vi "总磷流程.vi"   [LabVIEW 2016]
types:
  T1 = enum16{"步骤1", "步骤2", "步骤3", "步骤4", "步骤5", "步骤6", "步骤7", "步骤8", "步骤9", "步骤10"}
  T2 = enum32{"Bad", "Idle", "Run top level", "Running"}
  T3 = cluster{"因子编码":u32, "单位":u16, "标样参考值":sgl, "水样数据时间":timestamp, "水样实测值":sgl, "水样数据标识":string, "标样数据时间":timestamp, "标样实测值":sgl, "标样数据标识":string, "空白数据时间":timestamp, "空白实测值":sgl, "空白数据标识":string, "零点核查数据时间":timestamp, "零点核查实测值":sgl, "零点核查数据标识":string, "跨度核查数据时间":timestamp, "跨度核查实测值":sgl, "跨度核查数据标识":string, "加标回收数据时间":timestamp, "加标回收实测值":sgl, "加标回收数据标识":string, "平行样数据时间":timestamp, "平行样实测值":sgl, "平行样数据标识":string}
  T4 = cluster{"系统时间":timestamp, "工作状态":u16, "测量模式":u16, "告警代码":enum16{"无告警", "缺试剂告警", "缺水样告警", "缺蒸馏水告警", "缺标液告警", "仪表漏液告警", "标定异常告警", "超量程告警", "加热异常", "低试剂预警", "超上限告警", "超下限告警", "仪表内部其他异常", "滴定异常告警", "电极异常告警", "量程切换告警", "参数设置告警", "PH电极电位异常", "电导率电极异常", "浊度光度异常", "溶解氧电极异常", "溶解氧光强异常", "温度异常告警", "PH异常告警", "溶解氧异常告警", "电导率异常告警", "浊度异常告警", "叶绿素异常告警", "藻密度异常告警", "蓝绿藻异常告警", "ORP异常告警", "氨氮异常告警", "清洁刷异常告警", "SD卡异常告警", "蓝牙异常告警", "Wifi异常告警", "流程异常告警"}, "故障代码":enum16{"无故障", "电机故障", "温度故障", "通讯故障", "滴定故障"}, "日志代码":u16, "软件版本":u16, "F0":sgl, "F1":sgl, "F2":sgl, "F3":sgl, "T":sgl, "H":sgl, "id":u16, "flowid":u16, "量程":u16}
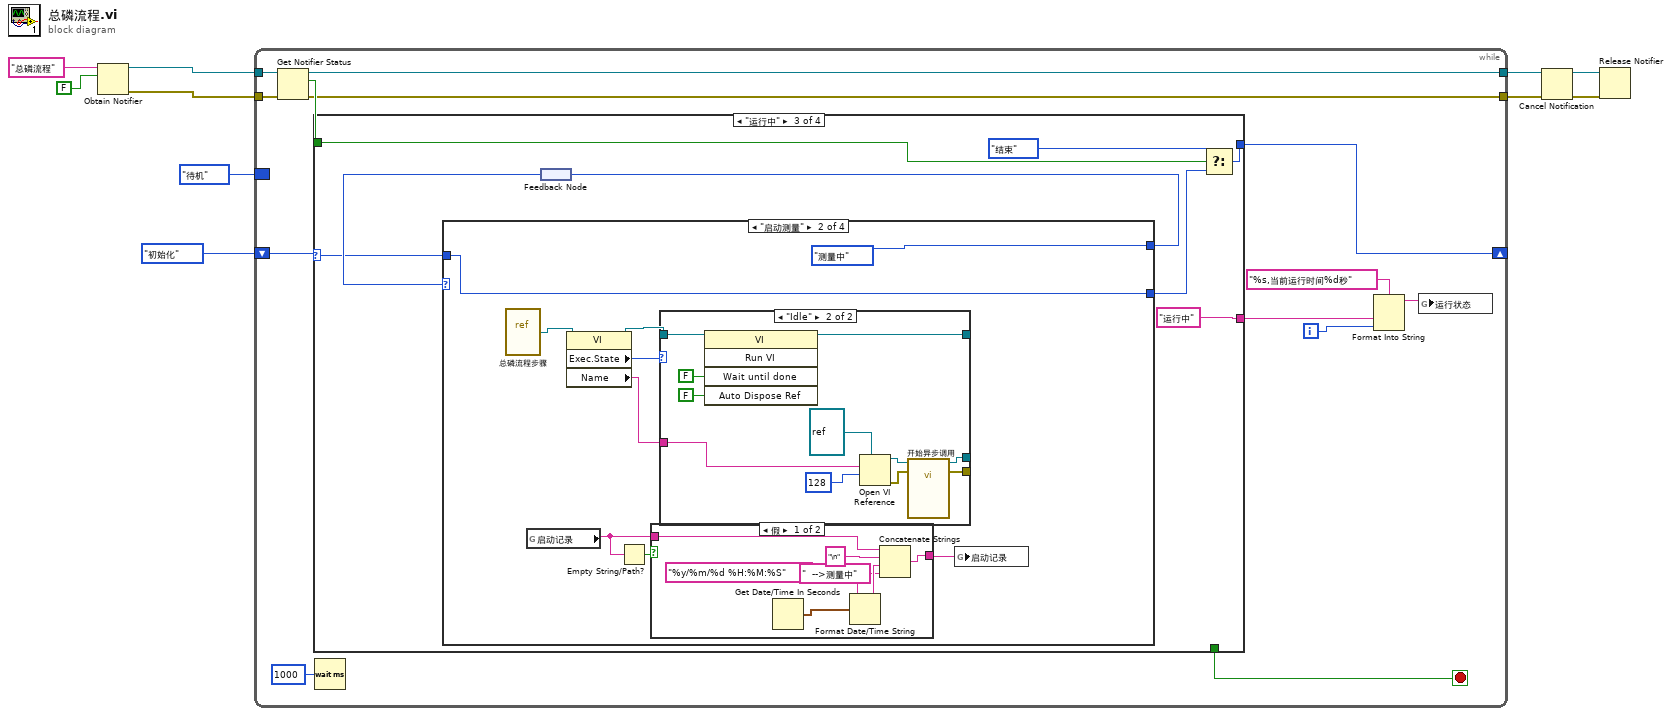
[diagram p0: block diagram]
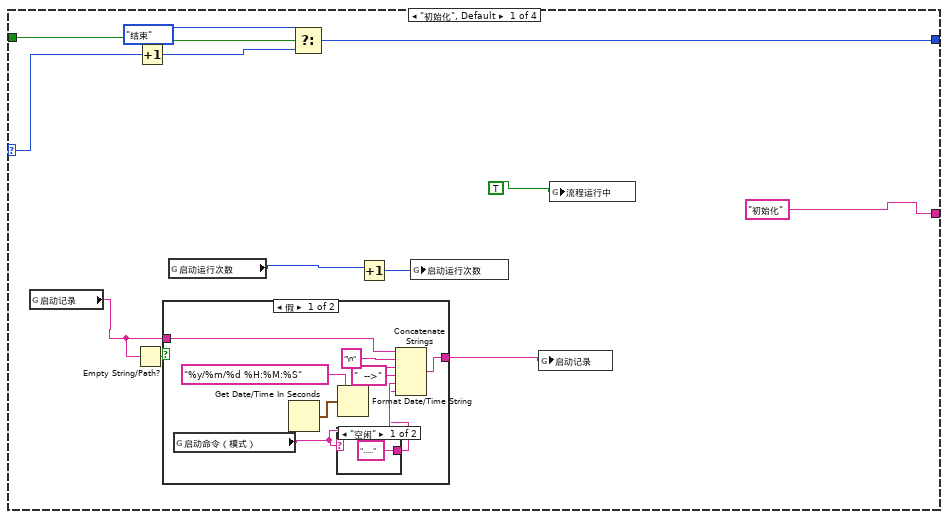
[diagram p2: hidden frame]
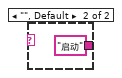
[diagram p3: hidden frame]
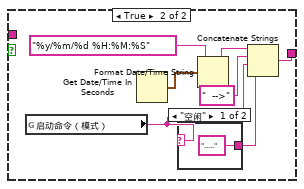
[diagram p4: hidden frame]
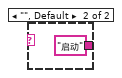
[diagram p5: hidden frame]
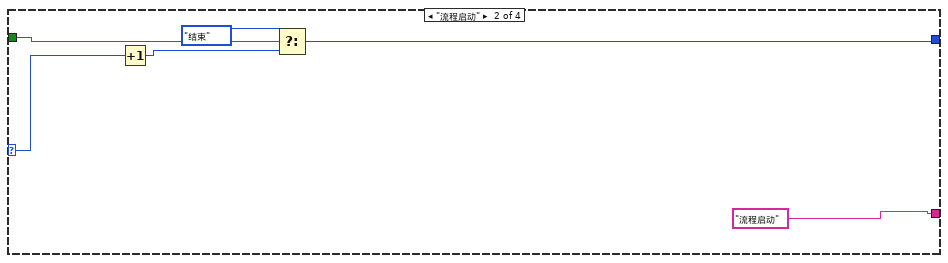
[diagram p6: hidden frame]
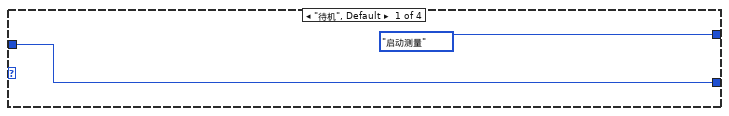
[diagram p7: hidden frame]
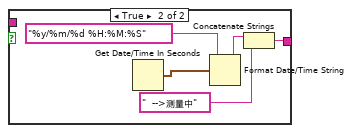
[diagram p8: hidden frame]
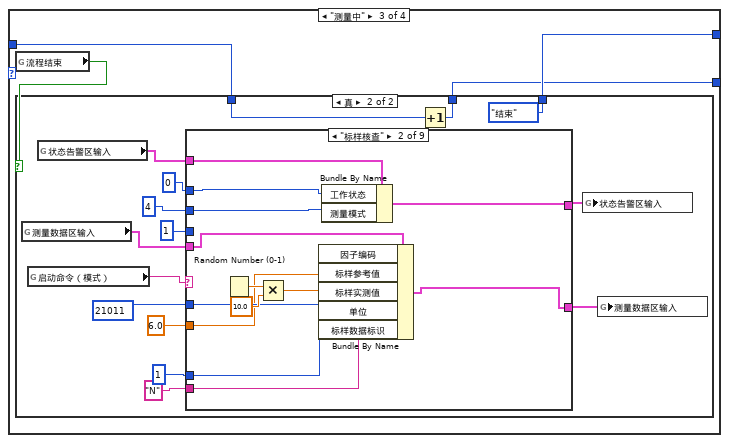
[diagram p10: hidden frame]
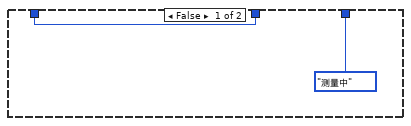
[diagram p11: hidden frame]
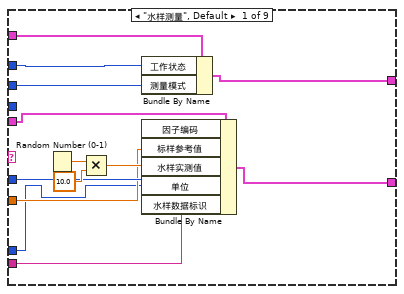
[diagram p12: hidden frame]
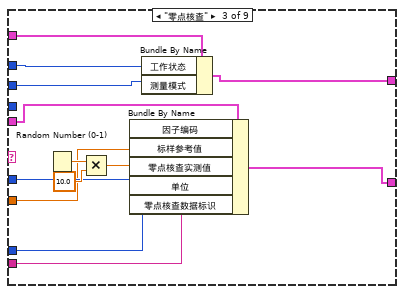
[diagram p13: hidden frame]
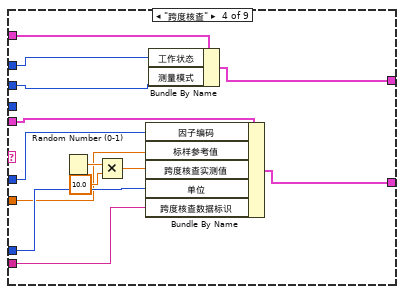
[diagram p14: hidden frame]
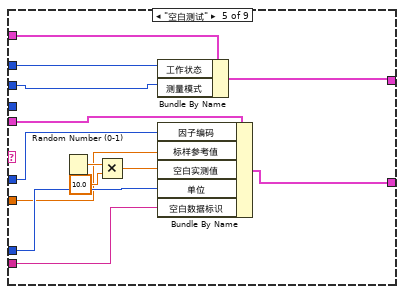
[diagram p15: hidden frame]
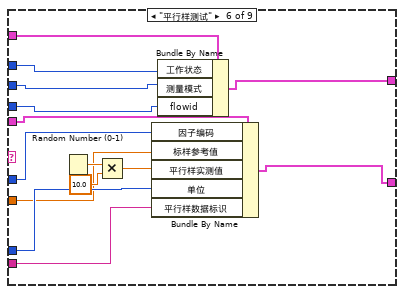
[diagram p16: hidden frame]
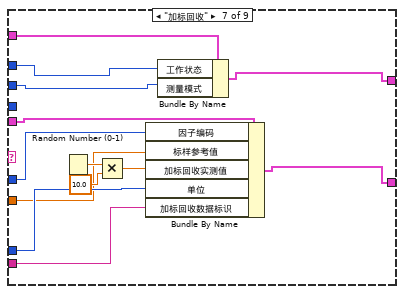
[diagram p17: hidden frame]
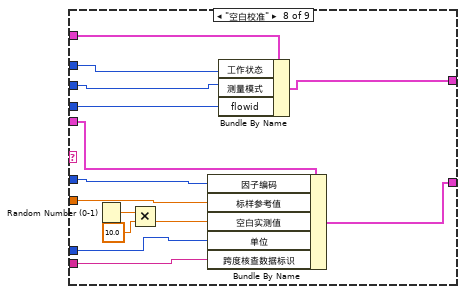
[diagram p18: hidden frame]
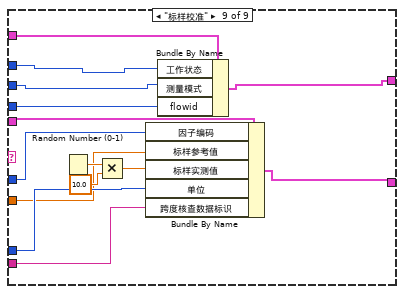
[diagram p19: hidden frame]
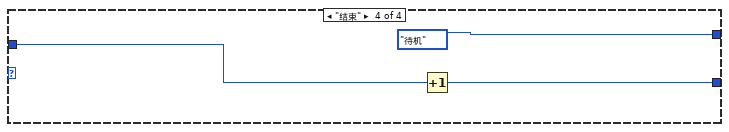
[diagram p20: hidden frame]
diagram:
  n1 = Obtain Notifier(name (unnamed)="总磷流程" ("名称（未命名）"), notification data type=FALSE) -> (notifier out=w7:refnum<notifier>, error out=w6:errorcluster)  [unwired: 2 in, 1 out]
  n2 = while {
    shift-right: [w20] -> _
    shift-left: enum16{"初始化", "流程启动", "运行中", "结束"}."初始化" ("枚举") -> [w23]
    tunnel: w7 -> [w15]
    tunnel: w6 -> [w14]
    tunnel: [w13] -> w5
    tunnel: [w12] -> w4
    border: enum16{"待机", "启动测量", "测量中", "结束"}."待机" -> [_]
    i -> [w18]
    stop <- w16 stop-if-true
    n3 = Get Notifier Status(notifier=w15, error in (no error)=w14) -> (notifier out=w13:refnum<notifier>, current notification=w21:bool, error out=w12:errorcluster)  [unwired: 2 out]
    n4 = case shown="\"运行中\"" w23 {
      selector: w23 -> [w33 w58 w64 w255]
      tunnel: [_ _ _ TRUE ("x")] -> w16
      tunnel: w21 -> [w35 w59 w68 _]
      tunnel: [w31 w57 w63 w255] -> w20
      tunnel: ["初始化" ("输入 1") "流程启动" ("输入 1") "运行中" ("输入 1") "结束" ("输入 1")] -> w17
      frame "初始化", Default {
        n5 = global read "总磷全局.vi" "启动记录"() -> (w25:string)
        n6 = Empty String/Path?(string/path=w25) -> (empty?=w29:bool)
        n7 = Increment(x=w33) -> (x+1=w32:enum16{"初始化", "流程启动", "运行中", "结束"})
        n8 = case shown="假" w29 {
          tunnel: w25 -> [w44 _]
          tunnel: [w39 w50] -> w24
          frame False {
            n9 = global read "总磷全局.vi" "启动命令（模式）"() -> (w37:string)
            n10 = Get Date/Time In Seconds() -> (seconds since 1Jan1904=w42:timestamp)
            n11 = case shown="\"空闲\"" w37 {
              tunnel: ["....." ("字符串") "启动" ("字符串")] -> w36
              frame "空闲" {
              }
              frame "", Default {
              }
            }
            n12 = Format Date/Time String(time format string (%c)="%y/%m/%d %H:%M:%S" ("时间格式字符串(%c)"), seconds (now)=w42) -> (date/time string=w40:string)  [unwired: 1 in]
            n13 = Concatenate Strings(w44, "\n" ("字符串"), w40, "  -->" ("字符串"), w37, w36) -> (w39:string)
          }
          frame True {
            n14 = global read "总磷全局.vi" "启动命令（模式）"() -> (w48:string)
            n15 = Get Date/Time In Seconds() -> (seconds since 1Jan1904=w53:timestamp)
            n16 = case shown="\"空闲\"" w48 {
              tunnel: ["....." ("字符串") "启动" ("字符串")] -> w47
              frame "空闲" {
              }
              frame "", Default {
              }
            }
            n17 = Format Date/Time String(time format string (%c)="%y/%m/%d %H:%M:%S" ("时间格式字符串(%c)"), seconds (now)=w53) -> (date/time string=w51:string)  [unwired: 1 in]
            n18 = Concatenate Strings(w51, "  -->" ("字符串"), w48, w47) -> (w50:string)
          }
        }
        n19 = global read "总磷全局.vi" "启动运行次数"() -> (w27:i32)
        n20 = Select(t=enum16{"初始化", "流程启动", "运行中", "结束"}."结束" ("枚举"), s=w35, f=w32) -> (s? t:f=w31:enum16{"初始化", "流程启动", "运行中", "结束"})
        n21 = Increment(x=w27) -> (x+1=w26:i32)
        n22 = global write "总磷全局.vi" "启动运行次数"(w26) -> ()
        n23 = global write "总磷全局.vi" "启动记录"(w24) -> ()
        n24 = global write "总磷全局.vi" "流程运行中"(TRUE ("流程运行中")) -> ()
      }
      frame "流程启动" {
        n25 = Increment(x=w58) -> (x+1=w60:enum16{"初始化", "流程启动", "运行中", "结束"})
        n26 = Select(t=enum16{"初始化", "流程启动", "运行中", "结束"}."结束" ("枚举"), s=w59, f=w60) -> (s? t:f=w57:enum16{"初始化", "流程启动", "运行中", "结束"})
      }
      frame "运行中" {
        n27 = feedback #1() -> (w67:enum16{"待机", "启动测量", "测量中", "结束"})
        n28 = case shown="\"启动测量\"" w67 {
          tunnel: [enum16{"待机", "启动测量", "测量中", "结束"}."启动测量" enum16{"待机", "启动测量", "测量中", "结束"}."测量中" w108 enum16{"待机", "启动测量", "测量中", "结束"}."待机"] -> w66
          tunnel: [w70 w79 w106 w247] -> w65
          tunnel: w64 -> [w70 w79 w107 w246]
          frame "待机", Default {
          }
          frame "启动测量" {
            n29 = vi-ref "总磷流程步骤.vi"() -> (w75:refnum<vi>)
            n30 = global read "总磷全局.vi" "启动记录"() -> (w73:string)
            n31 = property class="VI"(reference=w75) -> (reference out=w76:refnum<vi>, "Exec.State"=w77:T2, "Name"=w78:string)  [unwired: 1 in, 1 out]
            n32 = Empty String/Path?(string/path=w73) -> (empty?=w74:bool)
            n33 = case shown="假" w74 {
              tunnel: w73 -> [w87 _]
              tunnel: [w81 w88] -> w72
              frame False {
                n34 = Get Date/Time In Seconds() -> (seconds since 1Jan1904=w85:timestamp)
                n35 = Format Date/Time String(time format string (%c)="%y/%m/%d %H:%M:%S" ("时间格式字符串(%c)"), seconds (now)=w85) -> (date/time string=w83:string)  [unwired: 1 in]
                n36 = Concatenate Strings(w87, "\n" ("字符串"), w83, "  -->测量中" ("字符串")) -> (w81:string)
              }
              frame True {
                n37 = Get Date/Time In Seconds() -> (seconds since 1Jan1904=w92:timestamp)
                n38 = Format Date/Time String(time format string (%c)="%y/%m/%d %H:%M:%S" ("时间格式字符串(%c)"), seconds (now)=w92) -> (date/time string=w90:string)  [unwired: 1 in]
                n39 = Concatenate Strings(w90, "  -->测量中" ("字符串")) -> (w88:string)
              }
            }
            n40 = case shown="\"Idle\"" w77 {
              tunnel: w76 -> [w93 w101]
              tunnel: [w93 w102] -> _
              tunnel: w78 -> [_ w100]
              tunnel: [_ w95] -> _
              tunnel: [_ w94] -> _
              frame "Bad", Default {
              }
              frame "Idle" {
                n41 = invoke class="VI" method="Run VI"(reference=w101, "Wait until done"=FALSE ("结束前等待"), "Auto Dispose Ref"=FALSE ("自动销毁引用")) -> (reference out=w102:refnum<vi>)  [unwired: 2 in, 4 out]
                n42 = Open VI Reference(type specifier VI Refnum (for type only)=refnum<vi> refnum ("类型说明符VI引用句柄（仅用于类型）"), vi path=w100, options=128 ("选项")) -> (vi reference=w96:refnum<vi>, error out=w98:errorcluster)  [unwired: 3 in]
                n43 = call-by-ref "开始异步调用"(reference=w96, error in=w98) -> (reference out=w95:refnum<vi>, error out=w94:errorcluster)  [unwired: 12 in]
              }
            }
            n44 = global write "总磷全局.vi" "启动记录"(w72) -> ()
          }
          frame "测量中" {
            n45 = global read "总磷全局.vi" "流程结束"() -> (w105:bool)
            n46 = case shown="真" w105 {
              tunnel: [enum16{"待机", "启动测量", "测量中", "结束"}."测量中" enum16{"待机", "启动测量", "测量中", "结束"}."结束"] -> w108
              tunnel: w107 -> [w109 w118]
              tunnel: [w109 w117] -> w106
              frame False {
              }
              frame True {
                n47 = global read "总磷全局.vi" "测量数据区输入"() -> (w114:T3)
                n48 = global read "总磷全局.vi" "启动命令（模式）"() -> (w113:string)
                n49 = global read "总磷全局.vi" "状态告警区输入"() -> (w115:T4)
                n50 = case shown="\"标样核查\"" w113 {
                  tunnel: u32 21011 ("因子编码") -> [w133 w148 w161 w173 w186 w200 w213 w227 w241]
                  tunnel: u16 4 ("测量模式") -> [w134 w147 w160 w174 w187 w201 w214 w228 w242]
                  tunnel: sgl 6.0 ("标样参考值") -> [w132 w146 w159 w171 w184 w198 w211 w225 w239]
                  tunnel: u16 1 ("单位") -> [w131 w145 w158 w172 w185 w199 w212 w226 w240]
                  tunnel: "N" -> [w135 w144 w157 w170 w183 w197 w210 w224 w238]
                  tunnel: u16 0 ("工作状态") -> [w130 w143 w156 w169 w182 w196 w209 w223 w237]
                  tunnel: u16 1 ("工作状态") -> [_ _ _ _ _ w195 _ w222 w236]
                  tunnel: w114 -> [w129 w141 w153 w168 w179 w191 w207 w219 w233]
                  tunnel: [w128 w140 w152 w165 w178 w192 w205 w218 w232] -> w112
                  tunnel: w115 -> [w127 w142 w154 w167 w181 w194 w208 w221 w235]
                  tunnel: [w126 w139 w155 w166 w180 w193 w206 w220 w234] -> w111
                  frame "水样测量", Default {
                    n51 = Random Number (0-1)() -> (number: 0 to 1=w136:dbl)
                    n52 = Multiply(x=w136, y=10.0 ("数字(0-1)")) -> (x*y=w138:dbl)
                    n53 = Bundle By Name(cluster=w127, "工作状态"=w130, "测量模式"=w134) -> (w126:T4)
                    n54 = Bundle By Name(cluster=w129, "因子编码"=w133, "标样参考值"=w132, "水样实测值"=w138, "单位"=w131, "水样数据标识"=w135) -> (w128:T3)
                  }
                  frame "标样核查" {
                    n55 = Random Number (0-1)() -> (number: 0 to 1=w149:dbl)
                    n56 = Multiply(x=w149, y=10.0 ("数字(0-1)")) -> (x*y=w151:dbl)
                    n57 = Bundle By Name(cluster=w141, "因子编码"=w148, "标样参考值"=w146, "标样实测值"=w151, "单位"=w145, "标样数据标识"=w144) -> (w140:T3)
                    n58 = Bundle By Name(cluster=w142, "工作状态"=w143, "测量模式"=w147) -> (w139:T4)
                  }
                  frame "零点核查" {
                    n59 = Random Number (0-1)() -> (number: 0 to 1=w162:dbl)
                    n60 = Multiply(x=w162, y=10.0 ("数字(0-1)")) -> (x*y=w164:dbl)
                    n61 = Bundle By Name(cluster=w153, "因子编码"=w161, "标样参考值"=w159, "零点核查实测值"=w164, "单位"=w158, "零点核查数据标识"=w157) -> (w152:T3)
                    n62 = Bundle By Name(cluster=w154, "工作状态"=w156, "测量模式"=w160) -> (w155:T4)
                  }
                  frame "跨度核查" {
                    n63 = Random Number (0-1)() -> (number: 0 to 1=w175:dbl)
                    n64 = Multiply(x=w175, y=10.0 ("数字(0-1)")) -> (x*y=w177:dbl)
                    n65 = Bundle By Name(cluster=w168, "因子编码"=w173, "标样参考值"=w171, "跨度核查实测值"=w177, "单位"=w172, "跨度核查数据标识"=w170) -> (w165:T3)
                    n66 = Bundle By Name(cluster=w167, "工作状态"=w169, "测量模式"=w174) -> (w166:T4)
                  }
                  frame "空白测试" {
                    n67 = Random Number (0-1)() -> (number: 0 to 1=w188:dbl)
                    n68 = Multiply(x=w188, y=10.0 ("数字(0-1)")) -> (x*y=w190:dbl)
                    n69 = Bundle By Name(cluster=w181, "工作状态"=w182, "测量模式"=w187) -> (w180:T4)
                    n70 = Bundle By Name(cluster=w179, "因子编码"=w186, "标样参考值"=w184, "空白实测值"=w190, "单位"=w185, "空白数据标识"=w183) -> (w178:T3)
                  }
                  frame "平行样测试" {
                    n71 = Random Number (0-1)() -> (number: 0 to 1=w202:dbl)
                    n72 = Multiply(x=w202, y=10.0 ("数字(0-1)")) -> (x*y=w204:dbl)
                    n73 = Bundle By Name(cluster=w191, "因子编码"=w200, "标样参考值"=w198, "平行样实测值"=w204, "单位"=w199, "平行样数据标识"=w197) -> (w192:T3)
                    n74 = Bundle By Name(cluster=w194, "工作状态"=w196, "测量模式"=w201, "flowid"=w195) -> (w193:T4)
                  }
                  frame "加标回收" {
                    n75 = Random Number (0-1)() -> (number: 0 to 1=w215:dbl)
                    n76 = Multiply(x=w215, y=10.0 ("数字(0-1)")) -> (x*y=w217:dbl)
                    n77 = Bundle By Name(cluster=w207, "因子编码"=w213, "标样参考值"=w211, "加标回收实测值"=w217, "单位"=w212, "加标回收数据标识"=w210) -> (w205:T3)
                    n78 = Bundle By Name(cluster=w208, "工作状态"=w209, "测量模式"=w214) -> (w206:T4)
                  }
                  frame "空白校准" {
                    n79 = Random Number (0-1)() -> (number: 0 to 1=w229:dbl)
                    n80 = Multiply(x=w229, y=10.0 ("数字(0-1)")) -> (x*y=w231:dbl)
                    n81 = Bundle By Name(cluster=w219, "因子编码"=w227, "标样参考值"=w225, "空白实测值"=w231, "单位"=w226, "跨度核查数据标识"=w224) -> (w218:T3)
                    n82 = Bundle By Name(cluster=w221, "工作状态"=w223, "测量模式"=w228, "flowid"=w222) -> (w220:T4)
                  }
                  frame "标样校准" {
                    n83 = Random Number (0-1)() -> (number: 0 to 1=w243:dbl)
                    n84 = Multiply(x=w243, y=10.0 ("数字(0-1)")) -> (x*y=w245:dbl)
                    n85 = Bundle By Name(cluster=w233, "因子编码"=w241, "标样参考值"=w239, "标样实测值"=w245, "单位"=w240, "跨度核查数据标识"=w238) -> (w232:T3)
                    n86 = Bundle By Name(cluster=w235, "工作状态"=w237, "测量模式"=w242, "flowid"=w236) -> (w234:T4)
                  }
                }
                n87 = Increment(x=w118) -> (x+1=w117:enum16{"初始化", "流程启动", "运行中", "结束"})
                n88 = global write "总磷全局.vi" "状态告警区输入"(w111) -> ()
                n89 = global write "总磷全局.vi" "测量数据区输入"(w112) -> ()
              }
            }
          }
          frame "结束" {
            n90 = Increment(x=w246) -> (x+1=w247:enum16{"初始化", "流程启动", "运行中", "结束"})
          }
        }
        n91 = feedback-in #1(w66) -> ()
        n92 = Select(t=enum16{"初始化", "流程启动", "运行中", "结束"}."结束" ("枚举"), s=w68, f=w65) -> (s? t:f=w63:enum16{"初始化", "流程启动", "运行中", "结束"})
      }
      frame "结束" {
        w252 = FALSE ("流程结束")
        # "流程结束"
        n93 = global read "总磷全局.vi" "启动记录"() -> (w253:string)
        n94 = Empty String/Path?(string/path=w253) -> (empty?=w254:bool)
        n95 = case shown="真" w254 {
          tunnel: w253 -> [w264 _]
          tunnel: [w258 w265] -> w249
          frame False {
            n96 = Get Date/Time In Seconds() -> (seconds since 1Jan1904=w262:timestamp)
            n97 = Format Date/Time String(time format string (%c)="%y/%m/%d %H:%M:%S" ("时间格式字符串(%c)"), seconds (now)=w262) -> (date/time string=w260:string)  [unwired: 1 in]
            n98 = Concatenate Strings(w264, "\n" ("字符串"), w260, "  -->结束" ("字符串")) -> (w258:string)
          }
          frame True {
            n99 = Get Date/Time In Seconds() -> (seconds since 1Jan1904=w269:timestamp)
            n100 = Format Date/Time String(time format string (%c)="%y/%m/%d %H:%M:%S" ("时间格式字符串(%c)"), seconds (now)=w269) -> (date/time string=w267:string)  [unwired: 1 in]
            n101 = Concatenate Strings(w267, "  -->结束" ("字符串")) -> (w265:string)
          }
        }
        n102 = global write "总磷全局.vi" "启动记录"(w249) -> ()
        n103 = global write "总磷全局.vi" "步骤运行时间/秒"(0 ("运行时间/秒")) -> ()
        n104 = global write "总磷全局.vi" "当前步骤"(T1."步骤1" ("当前步骤 2")) -> ()
        n105 = global write "总磷全局.vi" "流程结束"(w252) -> ()
        n106 = global write "总磷全局.vi" "流程运行中"(w252) -> ()
      }
    }
    n107 = Wait (ms)(milliseconds to wait=u32 1000 ("等待时间（毫秒）")) -> ()  [unwired: 1 out]
    n108 = Format Into String(format string="%s,当前运行时间%d秒" ("格式字符串"), w17, w18) -> (resulting string=w11:string)  [unwired: 2 in, 1 out]
    n109 = global write "总磷全局.vi" "运行状态"(w11) -> ()
  }
  n110 = Cancel Notification(0:w5, 3:w4) -> (8:w3:refnum<notifier>, 11:w2:errorcluster)  [unwired: 1 out]
  n111 = Release Notifier(notifier=w3, error in (no error)=w2) -> ()  [unwired: 1 in, 3 out]
